vi "Script Custom Device.vi"(8 "error in":errorcluster, 9 "parameters configuration file path":path caption="path to parameters xml", 10 "hardware configuration file path":path, 11 "system definition path in":path) -> (0 "error out":errorcluster, 1 "Ballard MIL-STD 1553 custom device out":T1 format="%.0x", 2 "System Definition":refnum<k24>, 3 "system definition path out":path)   [LabVIEW 2023]
uses:
  <vilib>/NI/VeriStand Custom Device Testing Tools/VeriStandTestUtilities/VeriStandTestUtilities.lvlib
  Scripting/Ballard MIL-STD-1553 Scripting.lvlib
  Shared/Initialization Method.ctl
  Shared/Device Parameters.ctl
  <vilib>/NI VeriStand/Custom Device API/Custom Device Item Ref.ctl
  <vilib>/NI VeriStand/Custom Device API/Custom Device API.lvlib
  NationalInstruments.VeriStand.SystemDefinitionAPI
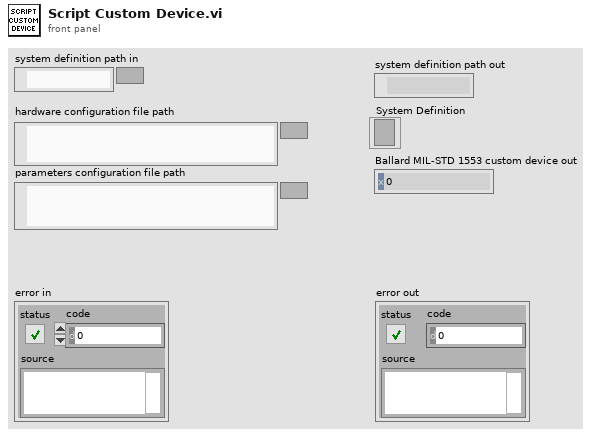
[diagram p1: front panel]
types:
  T1 = typedef "Custom Device API.lvlib/Custom Device Item Ref.ctl" = u64
  T2 = typedef "Device Parameters.ctl" = cluster{"initialization method":T3, "card number":i32, "PXI slot number":i32, "core number":i32}
  T3 = typedef "Initialization Method.ctl" = enum16{"PXI Slot Number", "Card Number"}
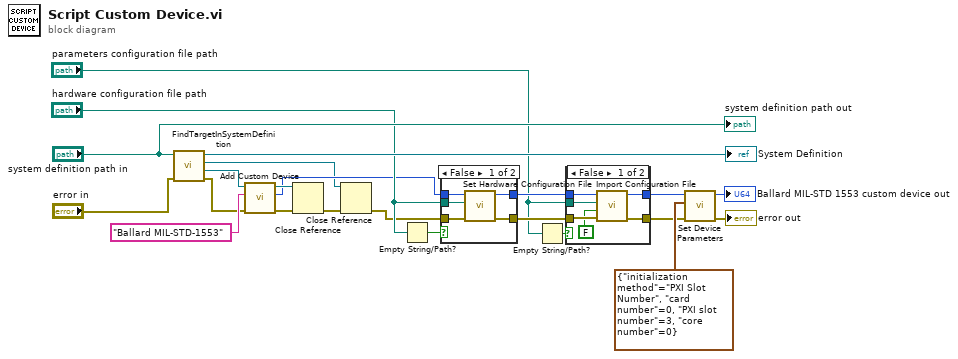
[diagram p0: block diagram]
diagram:
  n1 = call <vilib>:"FindTargetInSystemDefinition.vi"("error in"="error in", "system definition path"="system definition path in") -> ("error out"=w7:errorcluster, "Target"=w6:refnum<k24>, "Root"=w1:refnum<k24>, "System Definition"=→"System Definition":refnum<k24>)  [unwired: 6 in]
  n2 = call "Add Custom Device.vi"("error in"=w7, "name"="Ballard MIL-STD-1553", "target in"=w6) -> ("error out"=w23:errorcluster, "Ballard MIL-STD 1553 custom device"=w3:T1, "target out"=w4:refnum<k24>)  [unwired: 6 in]
  n3 = Close Reference(reference=w4, error in (no error)=w23) -> (error out=w5:errorcluster)
  n4 = Close Reference(reference=w1, error in (no error)=w5) -> (error out=w2:errorcluster)
  n5 = Empty String/Path?(string/path="hardware configuration file path") -> (empty?=w12:bool)
  n6 = case shown="False" w12 {
    tunnel: w2 -> [w28 w29]
    tunnel: w3 -> [w27 w30]
    tunnel: [w26 w29] -> w21
    tunnel: [w25 w30] -> w20
    tunnel: "hardware configuration file path" -> [w24 _]
    frame False {
      n7 = call "Set Hardware Configuration File.vi"("error in"=w28, "hardware configuration file path"=w24, "Ballard MIL-STD 1553 custom device in"=w27) -> ("error out"=w26:errorcluster, "Ballard MIL-STD 1553 custom device out"=w25:T1)  [unwired: 7 in]
    }
    frame True {
    }
  }
  n8 = Empty String/Path?(string/path="parameters configuration file path") -> (empty?=w10:bool)
  n9 = case shown="False" w10 {
    tunnel: w21 -> [w36 w37]
    tunnel: w20 -> [w35 w38]
    tunnel: [w34 w37] -> w18
    tunnel: [w33 w38] -> w17
    tunnel: "parameters configuration file path" -> [w32 _]
    frame False {
      n10 = call "Import Configuration File.vi"("error in"=w36, "create Tx/Rx folders for subaddresses?"=FALSE, "parameters configuration file path"=w32, "Ballard MIL-STD 1553 custom device in"=w35) -> ("error out"=w34:errorcluster, "Ballard MIL-STD 1553 custom device out"=w33:T1)  [unwired: 6 in]
    }
    frame True {
    }
  }
  n11 = call "Set Device Parameters.vi"("error in"=w18, "device parameters"=T2 {"initialization method"=enum."PXI Slot Number", "card number"=0, "PXI slot number"=3, "core number"=0}, "Ballard MIL-STD 1553 custom device in"=w17) -> ("error out"=→"error out":errorcluster, "Ballard MIL-STD 1553 custom device out"=→"Ballard MIL-STD 1553 custom device out":T1)  [unwired: 7 in]
  "system definition path out" <- "system definition path in"
